vi "PID_2Chan_V4_1loop_multiT_setVoltage.vi"() -> ()   [LabVIEW 2016]
uses:
  <vilib>/addons/control/pid/pid.llb/PID Advanced (DBL Array).vi
  <vilib>/addons/control/pid/pid.llb/PID Parameter Manager (DBL Array).vi
  <vilib>/addons/control/pid/pid.llb/PID Derivative Action Buffered (DBL Array).vi
  <vilib>/addons/control/pid/pid.llb/PID Get Advanced Error (DBL Array).vi
  <vilib>/addons/control/pid/pid.llb/PID Integral Action Buffered (DBL Array).vi
  <vilib>/addons/control/pid/pid.llb/PID Resize 1D Array.vi
  <vilib>/addons/control/pid/pid.llb/PID Get Advanced Error (DBL).vi
  <userlib>/Fluigent/Fluigent MFCS/FluigentMFCS_Full.llb/MFCS_EZ Detect.vi
  <userlib>/Fluigent/Fluigent MFCS/FluigentMFCS_Full.llb/MFCS_EZ Initialization.vi
  <userlib>/Fluigent/Fluigent MFCS/FluigentMFCS_Full.llb/MFCS_EZ Write Channel Pressure.vi
  <userlib>/Fluigent/Fluigent MFCS/FluigentMFCS_Full.llb/MFCS_EZ Set Channel EV.vi
  <userlib>/Fluigent/Fluigent MFCS/FluigentMFCS_Full.llb/MFCS_EZ Read All Channels Pressure.vi
  <userlib>/Fluigent/Fluigent MFCS/FluigentMFCS_Full.llb/MFCS_EZ Close.vi
  <vilib>/addons/control/pid/NI_PID_pid.lvlib
  <vilib>/Analysis/NI_AALBase.lvlib
  <vilib>/Analysis/baseanly.llb/Mean (DBL).vi
panel:
  in  "Set Voltage":dbl[](array[numeric])=[0.5, 0.5]
  out "Flow Rates":dbl[](array[numeric])=[219.92079825737392, 401.30921017675826]
  in  "FTot PID gains":cluster{"P":dbl, "I":dbl, "D":dbl}={"P"=0.03, "I"=0.0, "D"=0.0} {"D" format="%.3f"; "I" format="%.3f"; "P" format="%.7f"}
  in  "Ftot Setpoint":dbl=400.0
  in  "Vals to display":dbl=6000.0
  out "Flow plot":T1(graph)={"[0]"=219.92079825737392, "[1]"=401.30921017675826, "[2]"=220.0, "[3]"=400.0}
  out "Ferr":T2(graph)={"output[0]"=-0.03888029658961727, "output[1]"=-0.0396723140158781, "output[2]"=0.0}
  out "Pressures":dbl[](array[numeric])=[809.80517578125, 795.9191284179688]
  in  "F1 PID gains":cluster{"P":dbl, "I":dbl, "D":dbl} {"D" format="%.3f"; "I" format="%.3f"; "P" format="%.9f"}
  in  "reset Averging":bool
  in  "Set current Pressure\n to manual pressure":bool
  out "Pressures":cluster{"[0]":dbl, "[1]":dbl}(graph)={"[0]"=809.80517578125, "[1]"=795.9191284179688}
  in  "stop":bool
  in  "Valves":enum16{"1", "2", "3", "4", "5", "6", "7", "8"}[](array[ring])=[enum."6", enum."7"]
  in  "Pressure Channels":i16[](array[numeric])=[2, 3]
  in  "Manual Pressure Set":dbl[](array[numeric])=[810.792, 796.593]
  in  "PID On":bool
  in  "reinitialize? (F)":bool
  in  "F1 Setpoint":dbl=220.0
  in  "Add Ctrl?":bool
  in  "Boards":enum16{"A", "B", "C"}[](array[ring])=[enum."A", enum."A"]
  in  "Valves":enum16{"1", "2", "3", "4", "5", "6", "7", "8"}[](array[ring])=[enum."5", enum."4"]
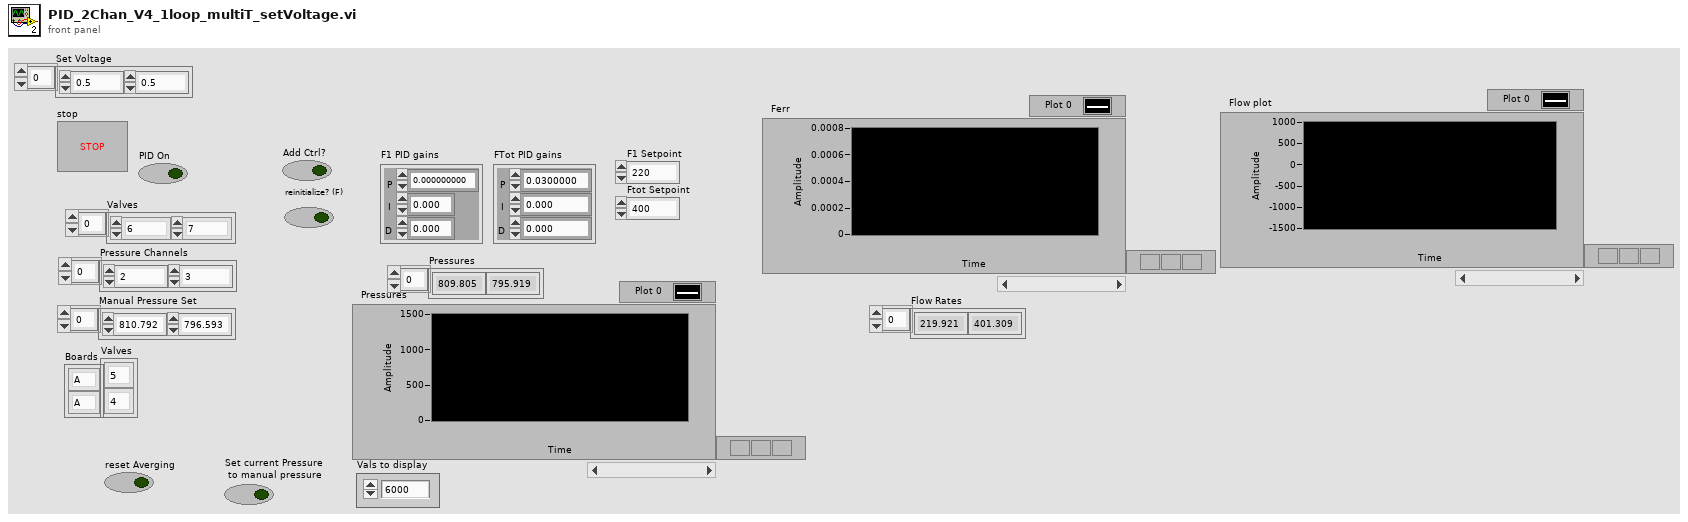
[diagram p1: front panel]
types:
  T1 = cluster{"[0]":dbl, "[1]":dbl, "[2]":dbl, "[3]":dbl}
  T2 = cluster{"output[0]":dbl, "output[1]":dbl, "output[2]":dbl}
  T3 = cluster{"setpoint high":dbl, "setpoint low":dbl}[]
  T4 = typedef "_EZmfcsSN.ctl" = u16
  T5 = typedef "_EZmfcsRefNum.ctl" = refnum<k1>
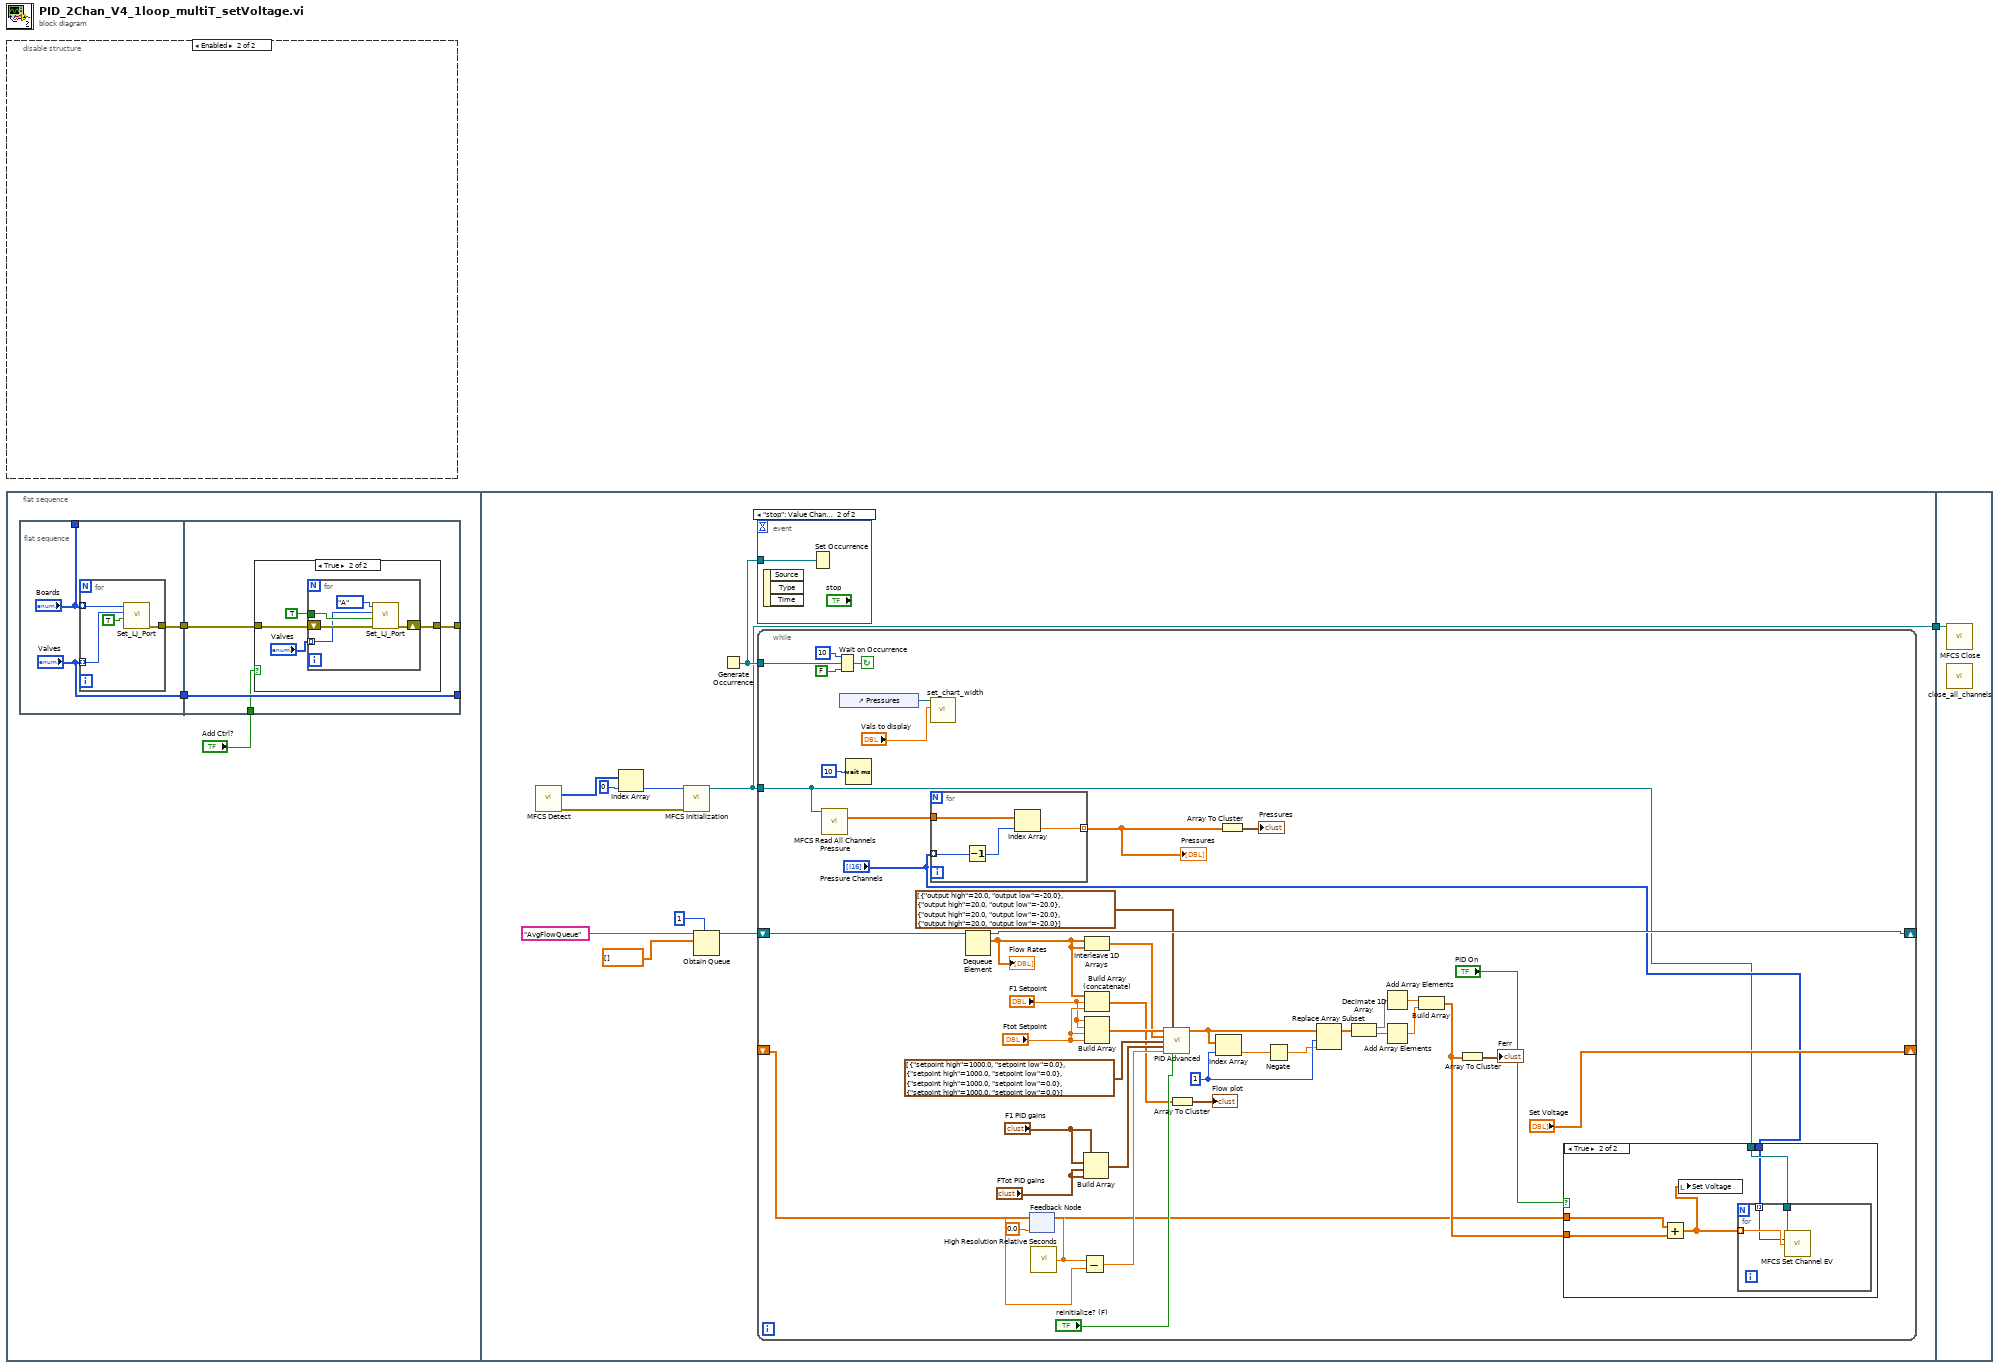
[diagram p0: block diagram]
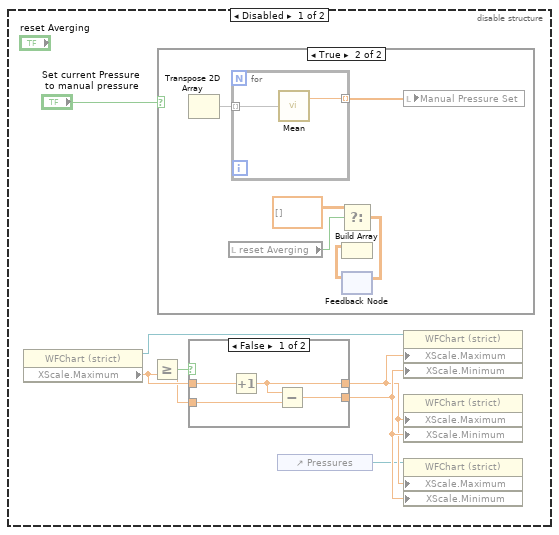
[diagram p2: hidden frame]
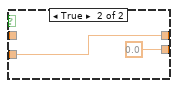
[diagram p3: hidden frame]
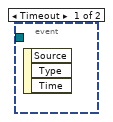
[diagram p6: hidden frame]
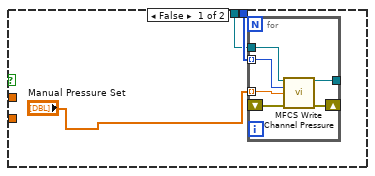
[diagram p7: hidden frame]
diagram:
  n1 = disable-structure shown="Enabled" {
    frame Disabled {
      n2 = property on="Property Node" class="WFChart (strict)"() -> (reference=w5:refnum<vi>, reference out=w6:refnum<vi>, "XScale.Maximum"=w4:dbl)  [unwired: 1 in, 1 out]
      n3 = Greater Or Equal?(y=w4) -> (x=w2:dbl, x >= y?=w3:bool)
      n4 = case shown="True" "Set current Pressure\n to manual pressure" {
        frame False {
        }
        frame True {
          n5 = Transpose 2D Array() -> (transposed array=w21:dbl[][])  [unwired: 1 in]
          n6 = local read "reset Averging"() -> (w22:bool)
          n7 = for {
            tunnel: w21 -> [w25] mode=indexing
            tunnel: [w24] -> w18 mode=indexing
            n8 = call-poly <vilib>:"Mean.vi"("X"=w25) -> ("mean"=w24:dbl)  [unwired: 1 out]
          }
          n9 = Select(t=dbl[][] [] ("appended array"), s=w22) -> (s? t:f=w19:dbl[][])  [unwired: 1 in]
          n10 = feedback-in #1(w19) -> ()
          n11 = feedback #1() -> (w23:dbl[][])  [unwired: 1 in]
          n12 = Build Array(w23) -> ()  [unwired: 1 in, 1 out]
          n13 = local write "Manual Pressure Set"(w18) -> ()
        }
      }
      n14 = case shown="False" w3 {
        tunnel: w2 -> [w13 w17]
        tunnel: w4 -> [w15 _]
        tunnel: [w12 w17] -> w9
        tunnel: [w14 0.0] -> w10
        frame False {
          n15 = Increment(x=w15) -> (x+1=w12:dbl)
          n16 = Subtract(x=w12, y=w13) -> (x-y=w14:dbl)
        }
        frame True {
        }
      }
      n17 = control-ref of="Pressures"() -> (w7:refnum<vi>)
      n18 = property on="Property Node" class="WFChart (strict)"(reference=w6, "XScale.Maximum"=w9, "XScale.Minimum"=w10) -> ()  [unwired: 1 in, 2 out]
      n19 = property on="Property Node" class="WFChart (strict)"("XScale.Maximum"=w9, "XScale.Minimum"=w10) -> (reference=w8:refnum<vi>)  [unwired: 1 in, 2 out]
      n20 = property on="Property Node" class="WFChart (strict)"(reference=w7, "XScale.Maximum"=w9, "XScale.Minimum"=w10) -> ()  [unwired: 1 in, 2 out]
    }
    frame Enabled {
    }
  }
  n21 = flat-sequence {
    tunnel: [w50] -> w1
    tunnel: w1 -> [w127]
    frame #0 {
      n22 = flat-sequence {
        tunnel: ["Boards"] -> _
        tunnel: [w31] -> w28
        tunnel: ["Valves"] -> w27
        tunnel: [w39] -> _
        tunnel: [w37] -> _
        tunnel: w28 -> [w38]
        tunnel: w27 -> [w39]
        tunnel: "Add Ctrl?" -> [w36]
        frame #0 {
          n23 = for {
            tunnel: "Valves" -> [w35] mode=indexing
            tunnel: "Boards" -> [w34] mode=indexing
            tunnel: [w32] -> w31
            n24 = call "Set_LJ_Port.vi"("State"=TRUE, "Channel"=w35, "Flowboard"=w34) -> ("error out"=w32:errorcluster)  [unwired: 8 in]
          }
        }
        frame #1 {
          n25 = case shown="True" w36 {
            tunnel: w38 -> [w40 w44]
            tunnel: [w40 w43] -> w37
            frame False {
            }
            frame True {
              n26 = for {
                tunnel: TRUE ("State") -> [w47]
                shift-right: [w48] -> w43
                shift-left: w44 -> [w49]
                tunnel: "Valves" -> [w46] mode=indexing
                n27 = call "Set_LJ_Port.vi"("error in"=w49, "State"=w47, "Channel"=w46, "Flowboard"=enum16{"A", "B", "C"}."A") -> ("error out"=w48:errorcluster)  [unwired: 7 in]
              }
            }
          }
        }
      }
    }
    frame #1 {
      n28 = call-poly <userlib>:"MFCS Detect.vi"() -> ("[SN MFCS_EZ]"=w59:T4[], "error out"=w57:errorcluster)  [unwired: 14 in]
      n29 = Index Array(array=w59, index=0) -> (element=w58:T4)
      n30 = call-poly <userlib>:"MFCS Initialization.vi"("SN MFCS_EZ"=w58, "error in (no error)"=w57) -> ("MFCS_EZ"=w50:T5)  [unwired: 11 in, 2 out]
      n31 = Obtain Queue(max queue size (-1, unlimited)=1, name (unnamed)="AvgFlowQueue", element data type=dbl[] [] ("appended array")) -> (queue out=w53:refnum<queue>)  [unwired: 2 in, 2 out]
      n32 = Generate Occurrence() -> (w52:refnum<k4>)
      n33 = event shown="[1] \"stop\": Value Change" {
        selector: _ -> [_ _]
        dyn-events: _ -> [_ _]
        timeout: _ -> [_ _]
        tunnel: w52 -> [_ w60]
        event Timeout {
          n34 = event-data() -> ()  [unwired: 1 in, 3 out]
        }
        event "stop": Value Change {
          n35 = event-data() -> ()  [unwired: 1 in, 3 out]
          n36 = Set Occurrence(w60) -> ()
        }
      }
      n37 = while {
        shift-right: [w104] -> _
        shift-left: w53 -> [w105]
        tunnel: w52 -> [w88]
        tunnel: w50 -> [w61]
        shift-right: ["Set Voltage"] -> _
        shift-left: _ -> [w63]
        stop <- w87 continue-if-true
        w96 = 1 ("index")
        n38 = call-poly <userlib>:"MFCS Read All Channels Pressure.vi"("MFCS_EZ"=w61) -> ("All Channels Pressure"=w69:dbl[])  [unwired: 12 in, 2 out]
        n39 = Wait on Occurrence(1:FALSE ("ignore previous (T)"), 2:w88, 3:10 ("ms timeout (-1)")) -> (0:w87:bool)
        n40 = control-ref of="Pressures"() -> (w68:refnum<vi>)
        n41 = Wait (ms)(milliseconds to wait=u32 10) -> ()  [unwired: 1 out]
        n42 = call "set_chart_width.vi"("Values to Display"="Vals to display", "Ref In"=w68) -> ()  [unwired: 10 in]
        n43 = for {
          tunnel: "Pressure Channels" -> [w108] mode=indexing
          tunnel: w69 -> [w109]
          tunnel: [w106] -> w65 mode=indexing
          n44 = Decrement(x=w108) -> (x-1=w107:i16)
          n45 = Index Array(array=w109, index=w107) -> (element=w106:dbl)
        }
        "Pressures" <- w65
        n46 = Dequeue Element(queue=w105) -> (queue out=w104:refnum<queue>, element=w74:dbl[])  [unwired: 2 in, 2 out]
        "Flow Rates" <- w74
        n47 = feedback #2(0.0 ("relative seconds")) -> (w100:dbl)
        n48 = call <vilib>:"High Resolution Relative Seconds.vi"() -> ("relative seconds"=w99:dbl)
        n49 = feedback-in #2(w99) -> ()
        n50 = Subtract(x=w99, y=w100) -> (x-y=w98:dbl)
        n51 = Build Array("F1 PID gains", "F1 PID gains", "FTot PID gains", "FTot PID gains") -> (w91:cluster{"P":dbl, "I":dbl, "D":dbl}[])
        n52 = Interleave 1D Arrays(w74, w74) -> (w73:dbl[])
        n53 = Build Array (concatenate)(w74, "F1 Setpoint", "Ftot Setpoint") -> (w78:dbl[])
        n54 = Build Array("F1 Setpoint", "F1 Setpoint", "Ftot Setpoint", "Ftot Setpoint") -> (w85:dbl[])
        n55 = call-poly <vilib>:"PID Advanced.vi"("setpoint"=w85, "output range"=cluster{"output high":dbl, "output low":dbl}[] [{"output high"=20.0, "output low"=-20.0}, {"output high"=20.0, "output low"=-20.0}, {"output high"=20.0, "output low"=-20.0}, {"output high"=20.0, "output low"=-20.0}], "process variable"=w73, "setpoint range"=T3 [{"setpoint high"=1000.0, "setpoint low"=0.0}, {"setpoint high"=1000.0, "setpoint low"=0.0}, {"setpoint high"=1000.0, "setpoint low"=0.0}, {"setpoint high"=1000.0, "setpoint low"=0.0}], "PID gains"=w91, "dt (s)"=w98, "reinitialize? (F)"="reinitialize? (F)") -> ("output"=w93:dbl[])  [unwired: 7 in, 1 out]
        n56 = Array To Cluster(array=w78) -> (cluster=→"Flow plot":T1)
        n57 = Index Array(array=w93, index=w96) -> (element=w95:dbl)
        n58 = Array To Cluster(array=w65) -> (cluster=→"Pressures":cluster{"[0]":dbl, "[1]":dbl})
        n59 = Negate(x=w95) -> (-x=w94:dbl)
        n60 = Replace Array Subset(array=w93, new element=w94, index=w96) -> (w83:dbl[])
        n61 = Decimate 1D Array(w83) -> (w82:dbl[], w81:dbl[])
        n62 = Add Array Elements(numeric array=w82) -> (sum=w80:dbl)
        n63 = Add Array Elements(numeric array=w81) -> (sum=w79:dbl)
        n64 = Build Array(w80, w79) -> (w70:dbl[])
        n65 = Array To Cluster(array=w70) -> (cluster=→"Ferr":cluster{"[0]":dbl, "[1]":dbl, "[2]":dbl})
        n66 = case shown="True" "PID On" {
          tunnel: w70 -> [_ w123]
          tunnel: w63 -> [_ w122]
          tunnel: "Pressure Channels" -> [w111 w120]
          tunnel: w61 -> [w110 w121]
          frame False {
            n67 = for {
              shift-right: [w117] -> _
              shift-left: _ -> [w118]
              tunnel: [w116] -> _
              tunnel: w111 -> [w115] mode=indexing
              tunnel: "Manual Pressure Set" -> [w114] mode=indexing
              tunnel: w110 -> [w113]
              n68 = call-poly <userlib>:"MFCS Write Channel Pressure.vi"("MFCS_EZ"=w113, "Channel Number (default=1)"=w115, "Pressure (mBar)"=w114, "error in (no error)"=w118) -> ("MFCS_EZ out"=w116:T5, "error out"=w117:errorcluster)  [unwired: 10 in]
            }
          }
          frame True {
            n69 = Add(x=w122, y=w123) -> (x+y=w119:dbl[])
            n70 = local write "Set Voltage"(w119) -> ()
            n71 = for {
              tunnel: w119 -> [w126] mode=indexing
              tunnel: w121 -> [w125]
              tunnel: w120 -> [w124] mode=indexing
              n72 = call-poly <userlib>:"MFCS Set Channel EV.vi"("MFCS_EZ"=w125, "Channel Number (0=All)"=w124, "% EV"=w126) -> ()  [unwired: 11 in, 2 out]
            }
          }
        }
      }
    }
    frame #2 {
      n73 = call-poly <userlib>:"MFCS Close.vi"("MFCS_EZ"=w127) -> ()  [unwired: 14 in, 1 out]
      n74 = call "close_all_channels.vi"() -> ()  [unwired: 12 in]
    }
  }
